vi "Swept Freq.vi"(7 "Sweep Start? (f)":bool, 8 "error in (no error)":errorcluster, 9 "Single? (f)":bool, 10 "ALC? (f)":bool, 11 "TxFrequencies":dbl[](array[numeric]) format="%.2f") -> (0 "error out":errorcluster, 1 "Tx Stat":T1, 2 "TxPower":dbl[](array[numeric]) format="%.2f", 3 "TxOn":bool[](array[boolean]))   [LabVIEW 2011]
uses:
  API/Controls/PIM.API.Command.Unique.ctl
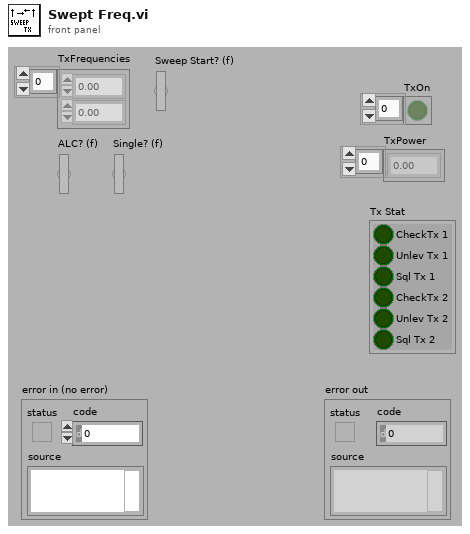
[diagram p1: front panel]
types:
  T1 = cluster{"CheckTx 1":bool, "Unlev Tx 1":bool, "Sql Tx 1":bool, "CheckTx 2":bool, "Unlev Tx 2":bool, "Sql Tx 2":bool}
  T2 = typedef "PIM.API.Command.Unique.ctl" = cluster{"#attributes":cluster{"Action":string}, "Double":dbl[], "Integer":i32[], "Boolean":bool[], "String":string[]}
  T3 = typedef "PIM.API.Response.Unique.ctl" = cluster{"#attributes":cluster{"Action":string, "Units":string}, "Double":dbl[], "Integer":i32[], "Boolean":bool[], "String":string[], "Sample":T4[], "Status":cluster{"#attributes":cluster{"Error":bool, "Code":i32}, "Message":string}[]}
  T4 = typedef "PIM.API.Response.Samples.ctl" = cluster{"TX1":cluster{"#attributes":cluster{"Frequency":dbl, "Power_dBm":dbl, "Power_Watts":dbl, "CheckTx":bool, "Unleveled":bool, "Squelched":bool, "Temperature":dbl, "ToneOn":bool}}, "TX2":cluster{"#attributes":cluster{"Frequency":dbl, "Power_dBm":dbl, "Power_Watts":dbl, "CheckTx":bool, "Unleveled":bool, "Squelched":bool, "Temperature":dbl, "ToneOn":bool}}, "IM":cluster{"#attributes":cluster{"Frequency":dbl, "Power_dBm":dbl, "PeakPower_dBm":dbl, "Power_dBc":dbl, "PeakPower_dBc":dbl, "IM_Order":u8, "IM Overload":bool}}[], "#attributes":cluster{"Count":u32, "Total":u32, "Finished?":bool, "Sweep Leg":T5, "F1":dbl, "F2":dbl, "FStep":dbl}}
  T5 = typedef "iQA Sweep Behavior.ctl" = enum16{"F2Down", "F1Up", "RxMultiIM"}
  T6 = cluster{"#attributes":cluster{"Error":bool, "Code":i32}, "Message":string}[]
  T7 = cluster{"#attributes":cluster{"Error":bool, "Code":i32}, "Message":string}
  T8 = cluster{"Boolean[0]":bool, "Boolean[1]":bool, "Boolean[2]":bool, "Boolean[3]":bool, "Boolean[4]":bool, "Boolean[5]":bool}
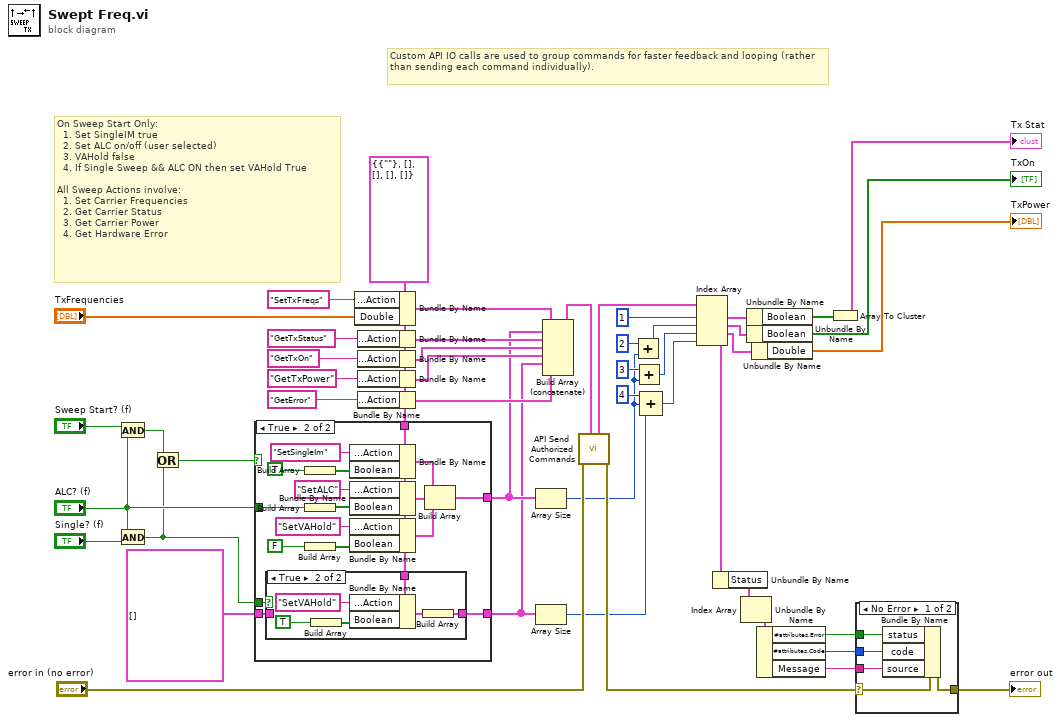
[diagram p0: block diagram]
diagram:
  w14 = T2 {"#attributes"={"Action"=""}, "Double"=[], "Integer"=[], "Boolean"=[], "String"=[]}
  # "On Sweep Start Only:\n  1. Set SingleIM true\n  2. Set ALC on/off (user selected)\n  3. VAHold false\n  4. If Single Sweep && ALC ON then set VAHold True\n\nAll Sweep Actions involve:\n  1. Set Carrier Frequencies\n  2. Get Carrier Status\n  3. Get Carrier Power\n  4. Get Hardware Error"
  # "Custom API IO calls are used to group commands for faster feedback and looping (rather than sending each command individually)."
  n1 = And(x="Sweep Start? (f)", y="ALC? (f)") -> (x .and. y?=w48:bool)
  n2 = And(x="ALC? (f)", y="Single? (f)") -> (x .and. y?=w3:bool)
  n3 = Or(x=w48, y=w3) -> (x .or. y?=w41:bool)
  n4 = case shown="True" w41 {
    tunnel: w14 -> [_ w54]
    tunnel: "ALC? (f)" -> [_ w60]
    tunnel: w3 -> [_ w53]
    tunnel: T2[] [] -> [w49 w52]
    tunnel: [w49 w51] -> w8
    tunnel: [w49 w50] -> w13
    frame False {
    }
    frame True {
      n5 = case shown="True" w53 {
        tunnel: w54 -> [_ w70]
        tunnel: [w67 w68] -> w51
        tunnel: w52 -> [w67 _]
        frame False {
        }
        frame True {
          n6 = Build Array(TRUE) -> (w69:bool[])
          n7 = Bundle By Name(cluster=w70, "#attributes.Action"="SetVAHold", "Boolean"=w69) -> (w71:T2)
          n8 = Build Array(w71) -> (w68:T2[])
        }
      }
      n9 = Build Array(TRUE) -> (w62:bool[])
      n10 = Build Array(w60) -> (w61:bool[])
      n11 = Build Array(FALSE) -> (w58:bool[])
      n12 = Bundle By Name(cluster=w54, "#attributes.Action"="SetSingleIm", "Boolean"=w62) -> (w57:T2)
      n13 = Bundle By Name(cluster=w54, "#attributes.Action"="SetALC", "Boolean"=w61) -> (w56:T2)
      n14 = Bundle By Name(cluster=w54, "#attributes.Action"="SetVAHold", "Boolean"=w58) -> (w55:T2)
      n15 = Build Array(w57, w56, w55) -> (w50:T2[])
    }
  }
  n16 = Bundle By Name(cluster=w14, "#attributes.Action"="SetTxFreqs", "Double"="TxFrequencies") -> (w32:T2)
  n17 = Bundle By Name(cluster=w14, "#attributes.Action"="GetTxStatus") -> (w31:T2)
  n18 = Bundle By Name(cluster=w14, "#attributes.Action"="GetTxOn") -> (w30:T2)
  n19 = Bundle By Name(cluster=w14, "#attributes.Action"="GetTxPower") -> (w17:T2)
  n20 = Bundle By Name(cluster=w14, "#attributes.Action"="GetError") -> (w16:T2)
  n21 = Array Size(array=w13) -> (size(s)=w6:i32)
  n22 = Array Size(array=w8) -> (size(s)=w5:i32)
  n23 = Build Array (concatenate)(w32, w13, w31, w30, w17, w8, w16) -> (w1:T2[])
  n24 = call "API Send Authorized Commands.vi"("Commands"=w1, "error in (no error)"="error in (no error)") -> ("error out"=w19:errorcluster, "Responses"=w2:T3[])  [unwired: 7 in, 1 out]
  n25 = Add(x=2 ("index"), y=w6) -> (x+y=w11:i32)
  n26 = Add(x=3 ("index"), y=w6) -> (x+y=w9:i32)
  n27 = Compound Arithmetic op=ADD(4 ("index"), w6, w5) -> (w4:i32)
  n28 = Index Array(array=w2, index #1=1 ("index"), index #2=w11, index #3=w9, index #4=w4) -> (element #1=w27:T3, element #2=w26:T3, element #3=w28:T3, element #4=w15:T3)
  n29 = Unbundle By Name(w15) -> ("Status"=w24:T6)
  n30 = Index Array(array=w24) -> (element=w23:T7)  [unwired: 1 in]
  n31 = Unbundle By Name(w27) -> ("Boolean"=w25:bool[])
  n32 = Unbundle By Name(w26) -> ("Boolean"=→"TxOn":bool[])
  n33 = Unbundle By Name(w28) -> ("Double"=→"TxPower":dbl[])
  n34 = Unbundle By Name(w23) -> ("#attributes.Error"=w22:bool, "#attributes.Code"=w21:i32, "Message"=w20:string)
  n35 = Array To Cluster(array=w25) -> (cluster=→"Tx Stat":T8)
  n36 = case shown="No Error" w19 {
    selector: w19 -> [w74 w79]
    tunnel: w22 -> [w78 _]
    tunnel: w21 -> [w77 _]
    tunnel: w20 -> [w76 _]
    tunnel: [w75 w79] -> w44
    frame No Error {
      n37 = Bundle By Name(cluster=w74, "status"=w78, "code"=w77, "source"=w76) -> (w75:errorcluster)
    }
    frame Error {
    }
  }
  "error out" <- w44
